vi "Get Identifier.vi"(8 "Error In":errorcluster, 11 "reference in":refnum<class "Camera.lvclass">) -> (0 "Error Out":errorcluster, 2 "Identifier":string, 3 "reference out":refnum<class "Camera.lvclass">)   [LabVIEW 2019, in "Camera.lvclass"]
uses:
  Camera.lvclass
  Interfaces/IConfigure/IConfigure.lvclass
  Interfaces/IConfiguration/IConfiguration.lvclass
  Camera.lvclass/Camera.ctl
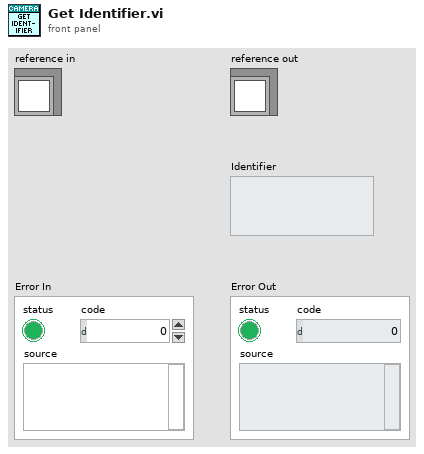
[diagram p1: front panel]
types:
  T1 = typedef "Camera.lvclass/ObjectAttributes.ctl" = cluster{"IConfigure":refnum<class "IConfigure.lvclass">, "Worker Enqueuer":refnum<class "Message Enqueuer.lvclass">, "Start Counter":i32, "Initialized":bool}
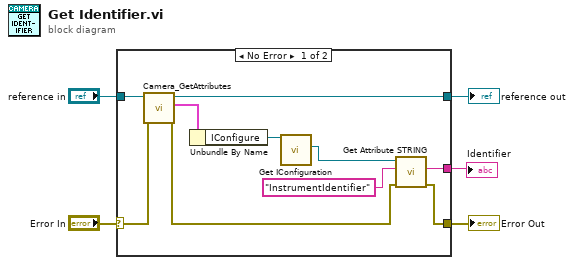
[diagram p0: block diagram]
diagram:
  n1 = case shown="No Error" "Error In" {
    selector: "Error In" -> [w15 w17]
    tunnel: [w7 w17] -> w4
    tunnel: [w12 w16] -> w2
    tunnel: "reference in" -> [w13 w16]
    tunnel: [w6 _] -> w1
    frame No Error {
      n2 = call "Camera_GetAttributes.vi"("Error In"=w15, "reference in"=w13) -> ("Error Out"=w8:errorcluster, "Data"=w14:T1, "reference out"=w12:refnum<class "Camera.lvclass">)  [unwired: 6 in, 1 out]
      n3 = Unbundle By Name(w14) -> ("IConfigure"=w11:refnum<class "IConfigure.lvclass">)
      n4 = call-dynamic "Get IConfiguration.vi"("IConfigure in"=w11) -> ("IConfiguration"=w10:refnum<class "IConfiguration.lvclass">)  [unwired: 9 in, 1 out]
      n5 = call-dynamic "Get Attribute STRING.vi"("error in"=w8, "Attribute"="InstrumentIdentifier", "IConfiguration in"=w10) -> ("error out"=w7:errorcluster, "Value"=w6:string)  [unwired: 6 in, 1 out]
    }
    frame Error {
    }
  }
  "Error Out" <- w4
  "reference out" <- w2
  "Identifier" <- w1
